vi "GraphADD.vi"(8 "错误输入（无错误）":errorcluster, 10 "曲线":cluster{dbl[], dbl[]}[](array[cluster]), 11 "XYGraph引用句柄":refnum<vi>) -> (0 "错误输出":errorcluster, 3 "引用输出":refnum<vi>)   [LabVIEW 2019]
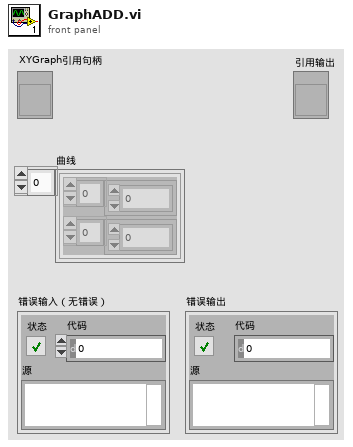
[diagram p1: front panel]
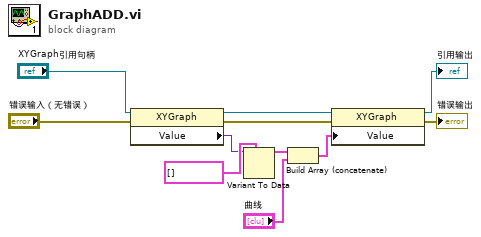
[diagram p0: block diagram]
diagram:
  n1 = property class="XYGraph"(reference="XYGraph引用句柄", error in="错误输入（无错误）") -> (reference out=w5:refnum<vi>, error out=w3:errorcluster, "Value"=w9:variant)
  n2 = Variant To Data(type=cluster{dbl[], dbl[]}[] [], Variant=w9) -> (data=w8:cluster{dbl[], dbl[]}[])  [unwired: 1 in, 1 out]
  n3 = Build Array (concatenate)(w8, "曲线") -> (w6:cluster{dbl[], dbl[]}[])
  n4 = property class="XYGraph"(reference=w5, error in=w3, "Value"=w6) -> (reference out=→"引用输出":refnum<vi>, error out=→"错误输出":errorcluster)
